vi "Import Scenario List.vi"(8 "error in (no error)":errorcluster, 11 "Node Ptr":u64 format="%.0x") -> (0 "error out":errorcluster)   [LabVIEW 2023, in "Vires VTD System Explorer.lvlib"]
uses:
  Vires VTD System Explorer.lvlib
  <vilib>/Utility/file.llb/Read Delimited Spreadsheet (string).vi
  Shared/Constants.vi
  <vilib>/NI VeriStand/Custom Device API/Set Item Property (String Array).vi
  <vilib>/NI VeriStand/Custom Device Tools/Custom Device Utility Library/Custom Device Utility Library.lvlib
  Shared/Vires VTD Shared.lvlib
  <vilib>/NI VeriStand/Custom Device API/Custom Device API.lvlib
panel:
  in  "Tag":string
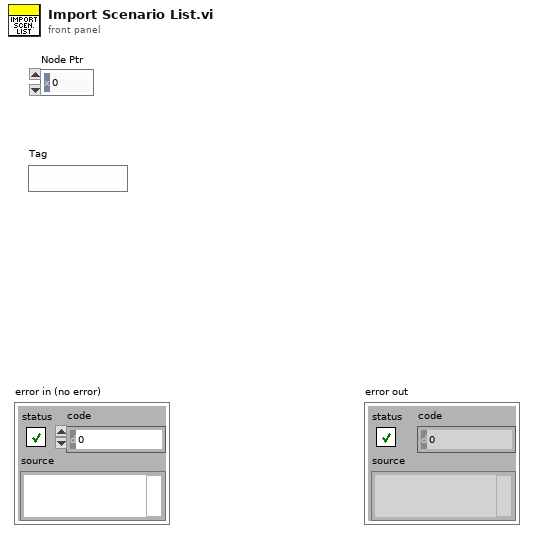
[diagram p1: front panel]
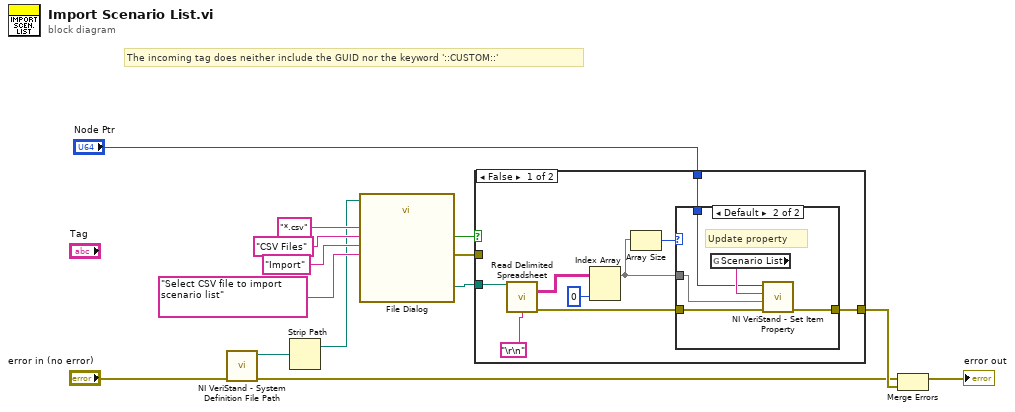
[diagram p0: block diagram]
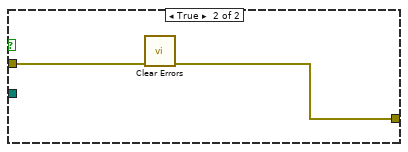
[diagram p3: hidden frame]
diagram:
  # "The incoming tag does neither include the GUID nor the keyword '::CUSTOM::'"
  n1 = call <vilib>:"NI VeriStand - System Definition File Path.vi"("error in (no error)"="error in (no error)") -> ("error out"=w5:errorcluster, "SDF path"=w6:path)  [unwired: 9 in]
  n2 = Strip Path(path=w6) -> (stripped path=w4:path)  [unwired: 1 out]
  n3 = call "File Dialog"("start path"=w4, "prompt"="Select CSV file to import scenario list", "button label"="Import", "pattern (all files)"="*.csv", "pattern label"="CSV Files") -> ("selected path"=w9:path, "cancelled"=w10:bool, "error out"=w8:errorcluster)  [unwired: 7 in, 1 out]
  n4 = case shown="False" w10 {
    tunnel: w9 -> [w23 _]
    tunnel: w8 -> [_ w31]
    tunnel: [w20 w30] -> w7
    tunnel: "Node Ptr" -> [w19 _]
    frame False {
      n5 = call-poly <vilib>:"Read Delimited Spreadsheet.vi"("file path (dialog if empty)"=w23, "delimiter (\\t)"="\r\n") -> ("all rows"=w18:string[][], "error out"=w21:errorcluster)  [unwired: 8 in, 4 out]
      n6 = Index Array(array=w18, index (col)=0 ("disabled index (col)")) -> (element=w16:string[])  [unwired: 1 in]
      n7 = Array Size(array=w16) -> (size(s)=w15:i32)
      n8 = case shown="Default" w15 {
        tunnel: w21 -> [w24 w28]
        tunnel: [w24 w27] -> w20
        tunnel: w19 -> [_ w26]
        tunnel: w16 -> [_ w25]
        frame 0 {
          # "no records found\n(Empty CSV?)\n>> do nothing"
        }
        frame Default {
          # "Update property"
          n9 = global read "Constants.vi" "Scenario List"() -> (w29:string)
          n10 = call-poly <vilib>:"NI VeriStand - Set Item Property.vi"("error in (no error)"=w28, "Value"=w25, "Property Name"=w29, "Item Ref in"=w26) -> ("error out"=w27:errorcluster)  [unwired: 5 in, 2 out]
        }
      }
    }
    frame True {
      n11 = call <vilib>:"Clear Errors.vi"("error in (no error)"=w31) -> ("error out"=w30:errorcluster)  [unwired: 5 in, 1 out]
    }
  }
  n12 = Merge Errors(w5, w7) -> (→"error out":errorcluster)
